vi "ManipChangeState.vi"(3 "Instruction String":string) -> (0 "Error Out":errorcluster, 1 "Advance Trigger":bool)   [LabVIEW 2019]
doc: "This VI changes the robot's master state.\n\nParameters:\n1. state --> the robot's master state number"
uses:
  SafeParser_Integer.vi
  constants.vi
  dsinstructions.vi
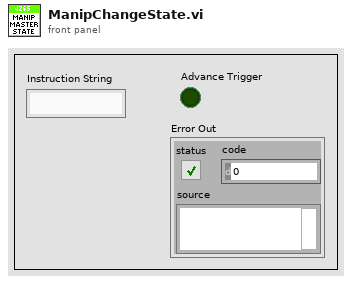
[diagram p1: front panel]
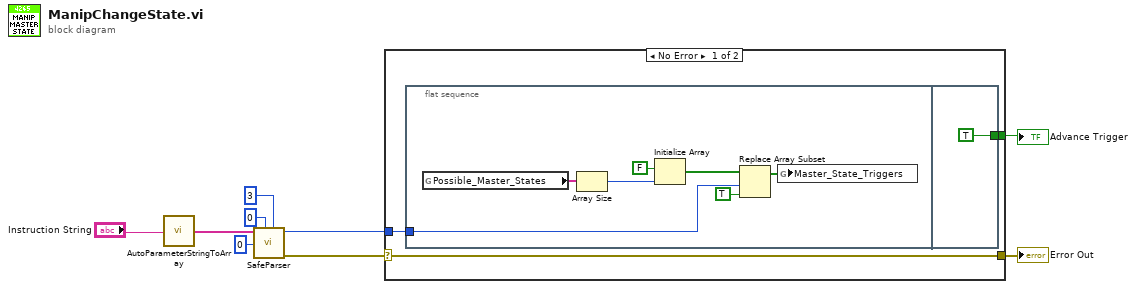
[diagram p0: block diagram]
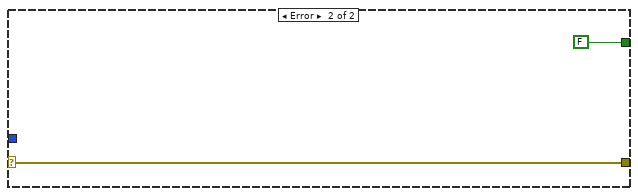
[diagram p2: hidden frame]
diagram:
  n1 = call "AutoParameterStringToArray.vi"("Parameter String"="Instruction String") -> ("Parsed Parameters"=w5:string[])
  n2 = call-poly "SafeParser.vi"("Maximum"=3, "Minimum"=0, "Array Index"=0 ("Parameter Index"), "String Array"=w5) -> ("Error Out"=w7:errorcluster, "Typecast  Value"=w1:i32)  [unwired: 6 in]
  n3 = case shown="No Error" w7 {
    selector: w7 -> [w11 w22]
    tunnel: [w12 FALSE ("Advance Trigger")] -> w9
    tunnel: [w11 w22] -> w8
    tunnel: w1 -> [w10 _]
    frame No Error {
      n4 = flat-sequence {
        tunnel: w10 -> [w13]
        tunnel: [TRUE ("Advance Trigger")] -> w12
        frame #0 {
          n5 = global read "constants.vi" "Possible_Master_States"() -> (w19:string[])
          n6 = Array Size(array=w19) -> (size(s)=w18:i32)
          n7 = Initialize Array(FALSE, w18) -> (w15:bool[])
          n8 = Replace Array Subset(array=w15, new element=TRUE ("new element/subarray"), index=w13) -> (w14:bool[])
          n9 = global write "dsinstructions.vi" "Master_State_Triggers"(w14) -> ()
        }
        frame #1 {
        }
      }
    }
    frame Error {
    }
  }
  "Advance Trigger" <- w9
  "Error Out" <- w8
